vi "crd_Acquire.vi"() -> ()   [LabVIEW 2011]
panel:
  in  "No Avg.":i32=1 min=1
  out "Decay":cluster{sgl[], "Best Exponential Fit":dbl[]}[](graph)
  out "error out":errorcluster
  out "Tau vs. T":dbl(graph)
  in  "stop":bool
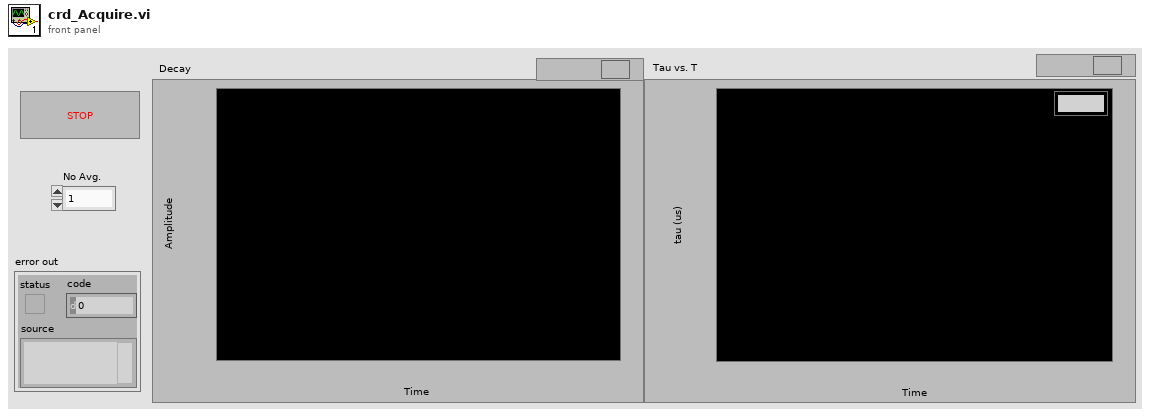
[diagram p1: front panel]
types:
  T1 = cluster{i32, "Sample Internal":sgl, "Data (Volts)":dbl[]}
  T2 = cluster{"Driver Version":string, "USB Version":string, "Hardware":string, "Variant":string, "Batch and Serial":string, "Cal Date":string, "Kernel Version":string, "Digital HW Version":string, "Analogue HW Version":string, "Firmware 1":string, "Firmware 2":string, "MSO":bool, "Number of Channels":i16}
  T3 = cluster{"Enabled":bool, "Coupling":i16, "Range":u16, "Analogue Offset":sgl}
  T4 = cluster{"preTriggerSamples":u32, "postTriggerSamples":u32, "timebase":u32, "Down-Sample Mode":i32, "Down Sample Ratio":u32, "Oversample":i16}
  T5 = cluster{"Trigger Enabled":bool, "Trigger Source":enum16{"Channel A", "Channel B", "Channel C", "Channel D", "Ext."}, "Trigger Threshold (Volts)":dbl, "Trigger Direction":u16, "Trigger Delay (samples)":u32, "Auto Trigger Time (ms)":i16}
  T6 = cluster{"Sample Frequency":sgl, "Sample Internal":sgl, "Max Samples Available":i32, "Number of Samples":u32, "Total Capture Time (sec) ":sgl, "Max Total Capture Time Available (sec)":sgl}
  T7 = cluster{"Channel D Buffer":i16[], "Channel C Buffer":i16[], "Channel B Buffer":i16[], "Channel A Buffer":i16[], "Port 0  Buffer ":i16[], "Port 1 Buffer ":i16[]}
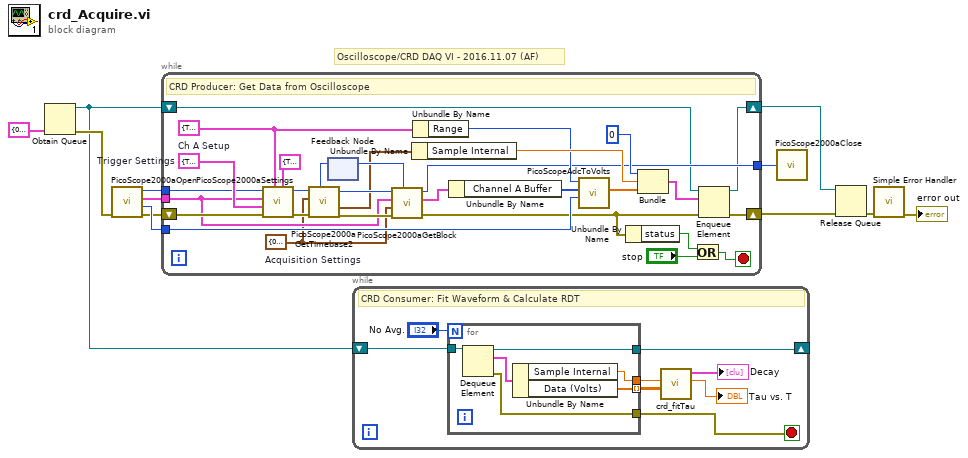
[diagram p0: block diagram]
diagram:
  # "Oscilloscope/CRD DAQ VI - 2016.11.07 (AF)"
  n1 = Obtain Queue(element data type=T1 {0, "Sample Internal"=8e-09, "Data (Volts)"=array[20000 elements]} ("Channel A 2")) -> (queue out=w4:refnum<queue>, error out=w7:errorcluster)  [unwired: 4 in, 1 out]
  n2 = call "PicoScope2000aOpen.vi"("error in (no error)"=w7) -> ("error out"=w11:errorcluster, "Max Adc value"=w12:i16, "Device Info"=w10:T2, "handle"=w9:i16)  [unwired: 7 in]
  n3 = while {
    tunnel: w10 -> [w25]
    tunnel: w9 -> [w34]
    tunnel: w12 -> [w32]
    tunnel: [w20] -> w3
    shift-right: [w18] -> w6
    shift-left: w4 -> [w15]
    shift-right: [w17] -> w5
    shift-left: w11 -> [w35]
    stop <- w41 stop-if-true
    w19 = T4 {"preTriggerSamples"=0, "postTriggerSamples"=10000, "timebase"=4, "Down-Sample Mode"=0, "Down Sample Ratio"=1, "Oversample"=1}  # Acquisition Settings
    w37 = T3 {"Enabled"=TRUE, "Coupling"=1, "Range"=5, "Analogue Offset"=0.0}  # Ch A Setup
    w36 = T5 {"Trigger Enabled"=TRUE, "Trigger Source"=enum."Channel B", "Trigger Threshold (Volts)"=0.0, "Trigger Direction"=3, "Trigger Delay (samples)"=0, "Auto Trigger Time (ms)"=1000}  # Trigger Settings
    # "CRD Producer: Get Data from Oscilloscope"
    n4 = call "PicoScope2000aSettings.vi"("Channel B Settings"=T3 {"Enabled"=TRUE, "Coupling"=0, "Range"=7, "Analogue Offset"=0.0}, "Channel A Settings"=w37, "error in"=w35, "Trigger Settings"=w36, "Device Info"=w25, "handle in"=w34) -> ("error out"=w30:errorcluster, "handle out"=w31:i16)  [unwired: 4 in]
    n5 = feedback #1() -> (w28:u32)  [unwired: 1 in]
    n6 = call "PicoScope2000aGetTimebase2.vi"("Number of Samples"=w28, "error in (no error)"=w30, "Acquisition Settings"=w19, "handle in"=w31) -> ("error out"=w27:errorcluster, "Properties Panel"=w24:T6, "handle out"=w26:i16)  [unwired: 5 in]
    n7 = call "PicoScope2000aGetBlock.vi"("error in"=w27, "Acquisition Settings"=w19, "Device Info"=w25, "handle in"=w26) -> ("error out"=w14:errorcluster, "Buffers (Max or non-aggregated)"=w23:T7, "handle out"=w20:i16, "noOfSamples"=w29:u32)  [unwired: 2 in, 2 out]
    n8 = feedback-in #1(w29) -> ()
    n9 = Unbundle By Name(w24) -> ("Sample Internal"=w38:sgl)
    n10 = Unbundle By Name(w37) -> ("Range"=w33:u16)
    n11 = Unbundle By Name(w23) -> ("Channel A Buffer"=w22:i16[])
    n12 = call "PicoScopeAdcToVolts.vi"("Max_adc"=w32, "Data"=w22, "Range Index"=w33) -> ("Data (Volts)"=w39:dbl[])  [unwired: 8 in]
    n13 = Unbundle By Name(w14) -> ("status"=w21:bool)
    n14 = Bundle(0, "Sample Internal"=w38, "Data (Volts)"=w39) -> (w16:T1)  [unwired: 1 in]
    n15 = Or(x=w21, y="stop") -> (x .or. y?=w41:bool)
    n16 = Enqueue Element(queue=w15, element=w16, error in (no error)=w14) -> (queue out=w18:refnum<queue>, error out=w17:errorcluster)  [unwired: 1 in, 1 out]
  }
  n17 = while {
    shift-right: [w44] -> _
    shift-left: w4 -> [w45]
    stop <- w43 stop-if-true
    # "CRD Consumer: Fit Waveform & Calculate RDT"
    n18 = for {
      N: "No Avg." -> [_]
      tunnel: [w56] -> w48
      tunnel: [w55] -> w47 mode=indexing
      tunnel: w45 -> [w54]
      tunnel: [w53] -> w44
      tunnel: [w51] -> w43
      n19 = Dequeue Element(queue=w54) -> (queue out=w53:refnum<queue>, element=w52:T1, error out=w51:errorcluster)  [unwired: 2 in, 1 out]
      n20 = Unbundle By Name(w52) -> ("Sample Internal"=w56:sgl, "Data (Volts)"=w55:dbl[])
    }
    n21 = call "crd_fitTau.vi"("y Data (volts)"=w47, "Sample Internal"=w48) -> ("tau (us)"=→"Tau vs. T":dbl, "Decay"=→"Decay":cluster{sgl[], "Best Exponential Fit":dbl[]}[])  [unwired: 8 in]
  }
  n22 = call "PicoScope2000aClose.vi"("handle"=w3) -> ()
  n23 = Release Queue(queue=w6, error in (no error)=w5) -> (error out=w1:errorcluster)  [unwired: 1 in, 2 out]
  n24 = call <vilib>:"Simple Error Handler.vi"("error in (no error)"=w1) -> ("error out"=→"error out":errorcluster)  [unwired: 4 in, 4 out]
